vi "Read Config File.vi"(8 "error in (no error)":errorcluster, 10 "Config File In":string) -> (0 "error out":errorcluster, 3 "Configuration out":T1)   [LabVIEW 2011, in "LVH-Build-Tools.lvlib"]
uses:
  LVH-Build-Tools.lvlib
  Type Defs/Configuration.ctl
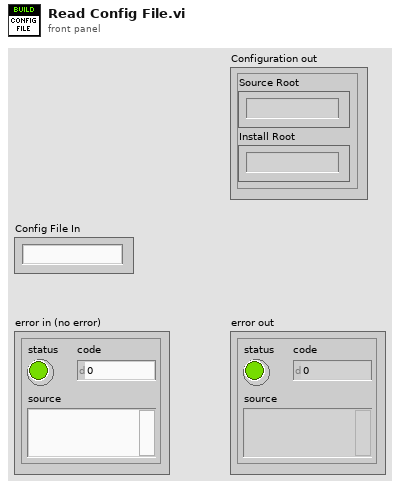
[diagram p1: front panel]
types:
  T1 = typedef "LVH-Build-Tools.lvlib/Configuration.ctl" = cluster{"Source Root":string, "Install Root":string, "Components":string[], "Ignore":string[]}
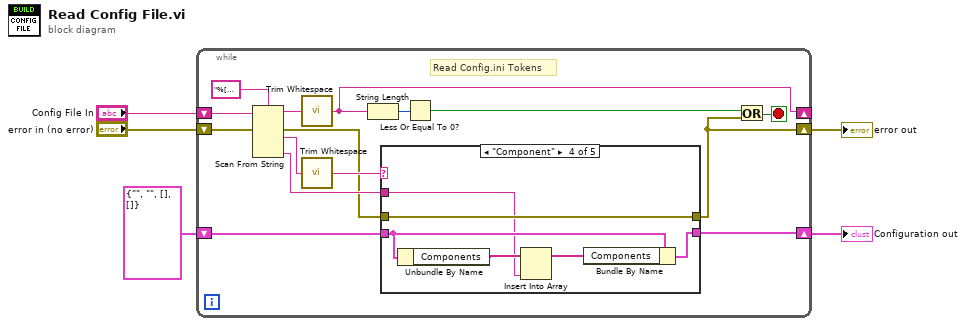
[diagram p0: block diagram]
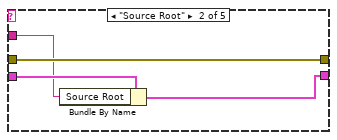
[diagram p3: hidden frame]
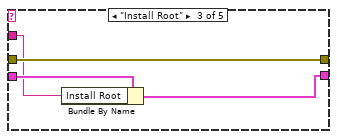
[diagram p4: hidden frame]
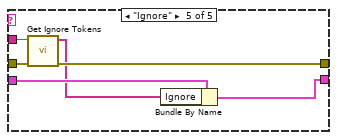
[diagram p5: hidden frame]
diagram:
  n1 = while {
    shift-right: [w10] -> _
    shift-left: "Config File In" -> [w19]
    shift-right: [w8] -> w4
    shift-left: "error in (no error)" -> [w18]
    shift-right: [w6] -> w5
    shift-left: T1 {"Source Root"="", "Install Root"="", "Components"=[], "Ignore"=[]} ("Configuration in") -> [w7]
    stop <- w14 stop-if-true
    # "Read Config.ini Tokens"
    n2 = Scan From String(format string="%[^=] %[=] %[^\n]", input string=w19, error in=w18) -> (remaining string=w11:string, error out=w9:errorcluster, output 1=w13:string, output 3=w16:string)  [unwired: 5 in, 1 out]
    n3 = call <vilib>:"Trim Whitespace.vi"("string"=w11) -> ("trimmed string"=w10:string)  [unwired: 1 in]
    n4 = call <vilib>:"Trim Whitespace.vi"("string"=w13) -> ("trimmed string"=w12:string)  [unwired: 1 in]
    n5 = String Length(string=w10) -> (length=w17:i32)
    n6 = case shown="\"Component\"" w12 {
      tunnel: w16 -> [_ w23 w27 w33 w42]
      tunnel: w9 -> [w22 w26 w30 w36 w41]
      tunnel: [w22 w26 w30 w36 w40] -> w8
      tunnel: [w21 w24 w29 w31 w38] -> w6
      tunnel: w7 -> [w21 w25 w28 w35 w39]
      frame Default {
      }
      frame "Source Root" {
        n7 = Bundle By Name(cluster=w25, "Source Root"=w23) -> (w24:T1)
      }
      frame "Install Root" {
        n8 = Bundle By Name(cluster=w28, "Install Root"=w27) -> (w29:T1)
      }
      frame "Component" {
        n9 = Unbundle By Name(w35) -> ("Components"=w34:string[])
        n10 = Insert Into Array(array=w34, new element=w33) -> (w32:string[])  [unwired: 1 in]
        n11 = Bundle By Name(cluster=w35, "Components"=w32) -> (w31:T1)
      }
      frame "Ignore" {
        n12 = call "Get Ignore Tokens.vi"("Error In"=w41, "Ignore String"=w42) -> ("ErrorOut"=w40:errorcluster, "Ignore Tokens"=w37:string[])  [unwired: 8 in]
        n13 = Bundle By Name(cluster=w39, "Ignore"=w37) -> (w38:T1)
      }
    }
    n14 = Less Or Equal To 0?(x=w17) -> (x <= 0?=w15:bool)
    n15 = Or(x=w15, y=w8) -> (x .or. y?=w14:bool)
  }
  "Configuration out" <- w5
  "error out" <- w4
